vi "Create Output Directory.vi"(6 "Local Data":T1, 8 "error in":errorcluster) -> (0 "error out":errorcluster, 4 "Local Data Out":T1)   [LabVIEW 2025]
uses:
  Controls/Local Data_Recording.ctl
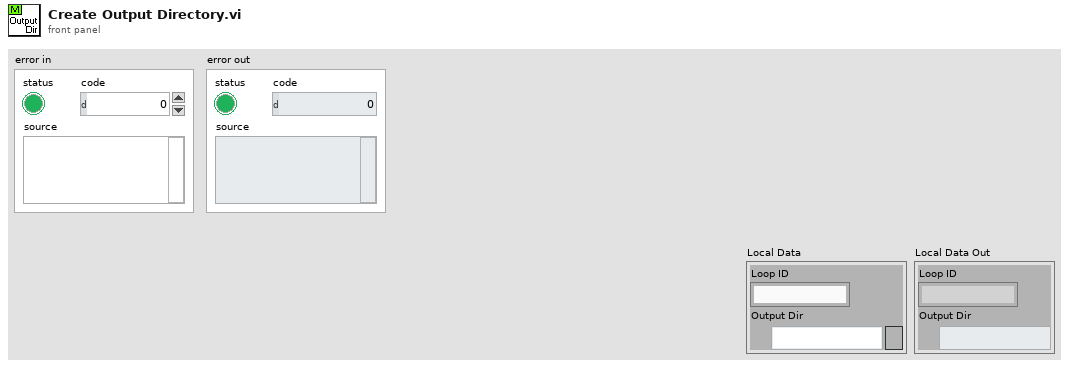
[diagram p1: front panel]
types:
  T1 = typedef "Local Data_Recording.ctl" = cluster{"Loop ID":string, "Output Dir":path}
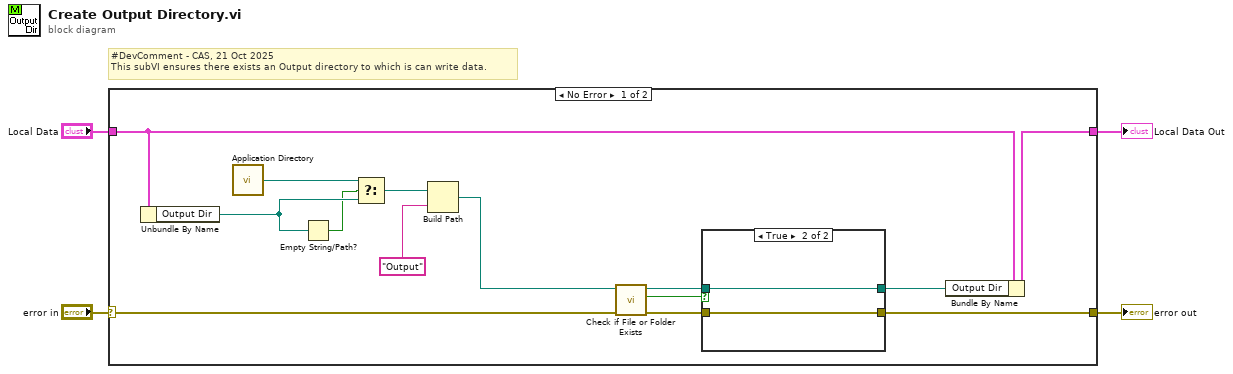
[diagram p0: block diagram]
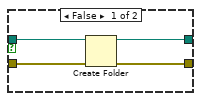
[diagram p2: hidden frame]
diagram:
  # "#DevComment - CAS, 21 Oct 2025\nThis subVI ensures there exists an Output directory to which is can write data."
  n1 = case shown="No Error" "error in" {
    selector: "error in" -> [w15 w26]
    tunnel: [w8 w26] -> w3
    tunnel: "Local Data" -> [w7 w25]
    tunnel: [w5 w25] -> w1
    frame No Error {
      n2 = Unbundle By Name(w7) -> ("Output Dir"=w17:path)
      n3 = call <vilib>:"Application Directory.vi"() -> ("Application Directory"=w18:path)
      n4 = Empty String/Path?(string/path=w17) -> (empty?=w16:bool)
      n5 = Select(t=w18, s=w16, f=w17) -> (s? t:f=w14:path)
      n6 = Build Path(base path=w14, name or relative path="Output") -> (appended path=w12:path)
      n7 = call <vilib>:"Check if File or Folder Exists.vi"("error in (no error)"=w15, "path"=w12) -> ("error out"=w10:errorcluster, "file or folder exists?"=w9:bool, "dup path"=w11:path)  [unwired: 7 in]
      n8 = case shown="True" w9 {
        tunnel: w11 -> [w21 w23]
        tunnel: w10 -> [w22 w24]
        tunnel: [w20 w24] -> w8
        tunnel: [w19 w23] -> w6
        frame False {
          n9 = Create Folder(path (use dialog)=w21, error in=w22) -> (created path=w19:path, error out=w20:errorcluster)  [unwired: 1 in, 1 out]
        }
        frame True {
        }
      }
      n10 = Bundle By Name(cluster=w7, "Output Dir"=w6) -> (w5:T1)
    }
    frame Error {
    }
  }
  "error out" <- w3
  "Local Data Out" <- w1
